vi "ReadOneChannel.vi"(4 "error in (no error)":errorcluster, 7 "Circuit ID":i32=1038 format="%_4g") -> (0 "Error out":errorcluster, 3 "OneChannelsValue":dbl)   [LabVIEW 2009]
doc: "Issues a SCPI read to one channel of the 34980 DMM"
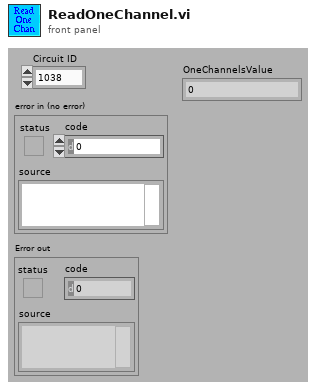
[diagram p1: front panel]
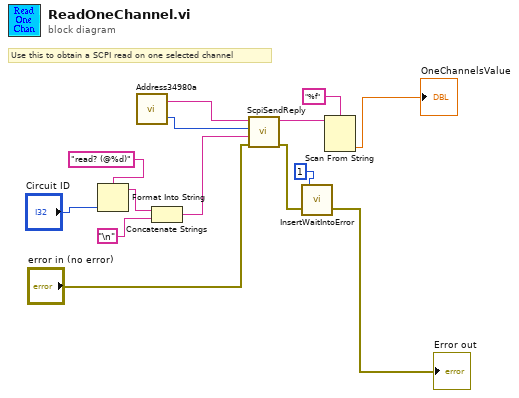
[diagram p0: block diagram]
diagram:
  # "Use this to obtain a SCPI read on one selected channel"
  n1 = Format Into String(format string="read? (@%d)", "Circuit ID") -> (resulting string=w7:string)  [unwired: 2 in, 1 out]
  n2 = call "Address34980a.vi"() -> ("Port"=w11:i32, "IP address"=w10:string)  [unwired: 2 in]
  n3 = Concatenate Strings(w7, "\n") -> (w5:string)
  n4 = call "ScpiSendReply.vi"("error in (no error)"="error in (no error)", "Command"=w5, "TCP port"=w11, "IP Address"=w10) -> ("Error out"=w4:errorcluster, "Reply"=w13:string)  [unwired: 5 in]
  n5 = call "InsertWaitIntoError.vi"("error in (no error)"=w4, "Wait (msecs)"=1) -> ("error out"=→"Error out":errorcluster)  [unwired: 1 in]
  n6 = Scan From String(format string="%f", input string=w13) -> (output 1=→"OneChannelsValue":dbl)  [unwired: 3 in, 3 out]
